vi "Freefield-Save data.vi"(0 "Mag":dbl[](array[numeric]), 5 "Phase":dbl[](array[numeric]), 7 "Frequency":dbl[](array[numeric]), 9 "Stimulus":T1={"Min Freq (Hz)"=1000.0, "Max Freq (Hz)"=50000.0, "Freq Step (Hz)"=50.0, "Waveform"=enum."Chirp", "Attenuation (dB)"=30.0, "Sample Rate (Hz)"=100000.0}, 11 "error in (no error)":errorcluster, 12 "Speaker":string, 13 "Rig":string) -> (6 "new file path":path, 15 "error out":errorcluster)   [LabVIEW 2020]
uses:
  In-Ear Calibration VIs/LV Source/Type Defs/Cal Stimulus.ctl
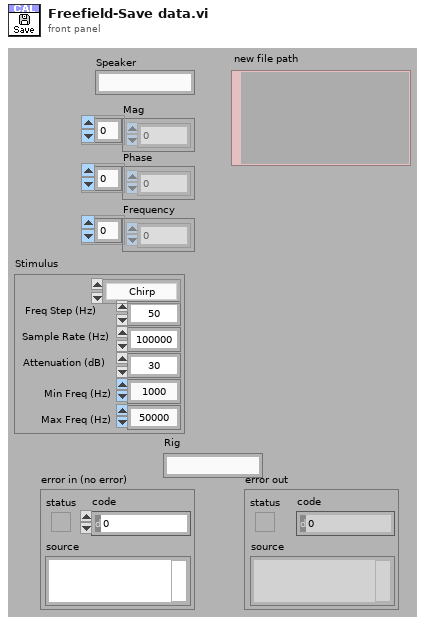
[diagram p1: front panel]
types:
  T1 = typedef "Cal Stimulus.ctl" = cluster{"Min Freq (Hz)":dbl, "Max Freq (Hz)":dbl, "Freq Step (Hz)":dbl, "Waveform":enum16{"Chirp", "Weighted"}, "Attenuation (dB)":dbl, "Sample Rate (Hz)":dbl}
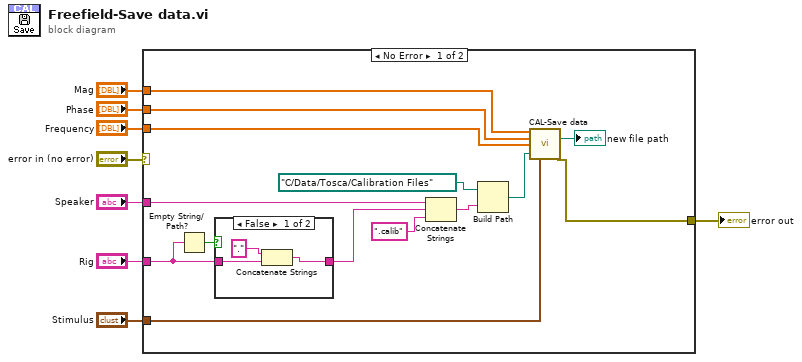
[diagram p0: block diagram]
diagram:
  n1 = case shown="No Error" "error in (no error)" {
    selector: "error in (no error)" -> [_ w27]
    tunnel: "Phase" -> [w21 _]
    tunnel: "Mag" -> [w20 _]
    tunnel: "Frequency" -> [w22 _]
    tunnel: "Speaker" -> [w14 _]
    tunnel: [w18 w27] -> w3
    tunnel: "Stimulus" -> [w12 _]
    tunnel: "Rig" -> [w9 _]
    frame No Error {
      n2 = Empty String/Path?(string/path=w9) -> (empty?=w11:bool)
      n3 = case shown="False" w11 {
        tunnel: w9 -> [w25 w26]
        tunnel: [w24 w26] -> w10
        frame False {
          n4 = Concatenate Strings("." ("string"), w25) -> (w24:string)
        }
        frame True {
        }
      }
      n5 = Concatenate Strings(w14, w10, ".calib" ("string")) -> (w16:string)
      n6 = Build Path(base path=path "C:/Data/Tosca/Calibration Files", name or relative path=w16) -> (appended path=w15:path)
      n7 = call "CAL-Save data.vi"("Mag"=w20, "Phase"=w21, "Frequency"=w22, "path"=w15, "Cal Stimulus"=w12) -> ("new file path"=→"new file path":path, "error out"=w18:errorcluster)  [unwired: 9 in]
    }
    frame Error {
    }
  }
  "error out" <- w3
